vi "SmartSEM Remote API FIB Gun Valve.vi"(5 "Wait (ms)":u32=2000, 7 "Iterations":u32=3, 8 "error in":errorcluster, 10 "FIB Gun Valve":enum16{"Close", "Open"}(ring), 11 "Api":refnum<k7>(container)) -> (0 "error out":errorcluster, 3 "Api out":refnum<k7>)   [LabVIEW 2018]
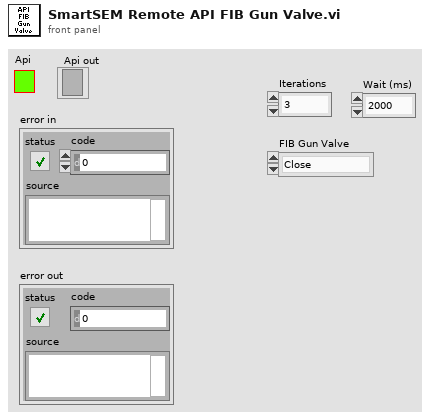
[diagram p1: front panel]
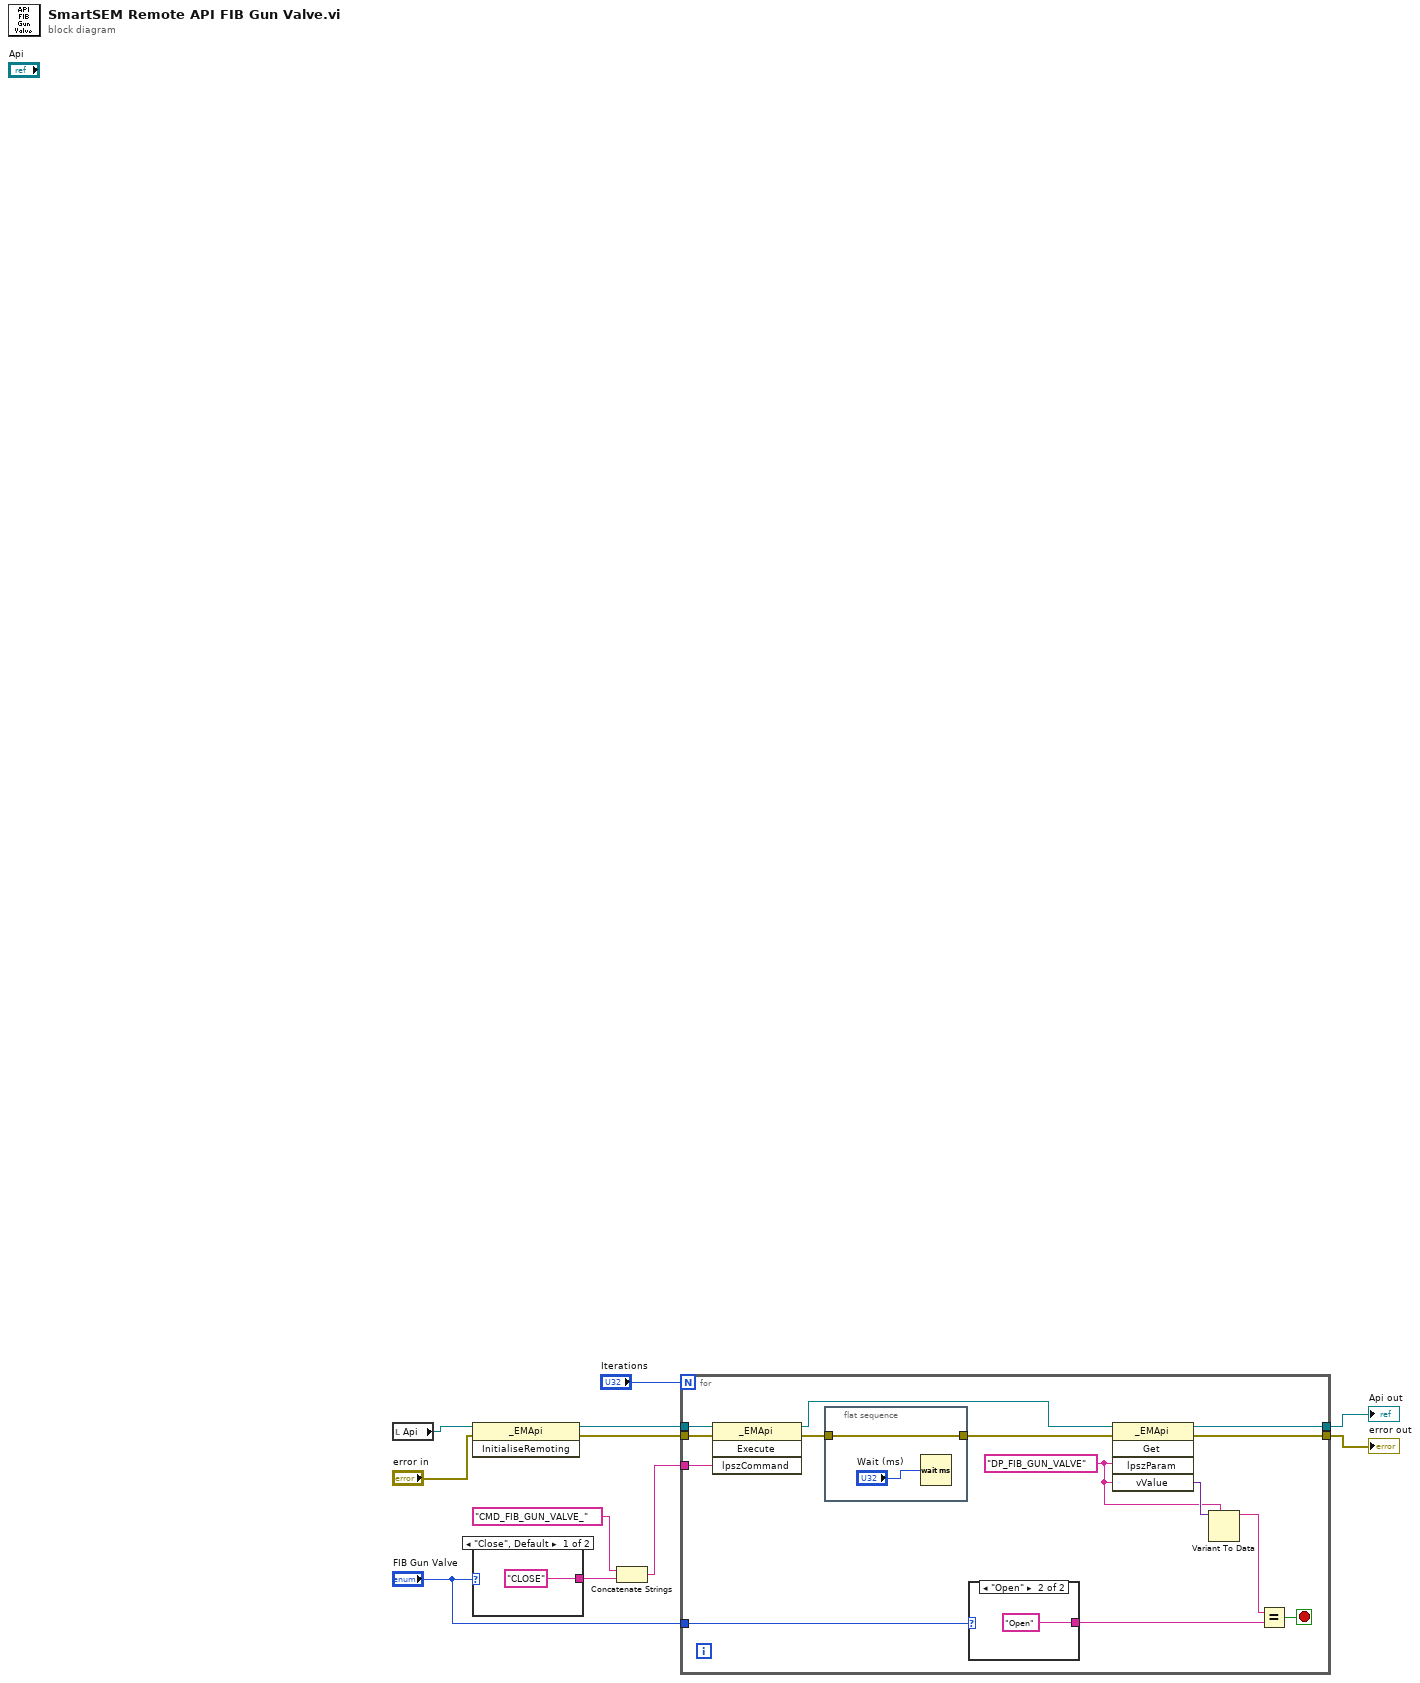
[diagram p0: block diagram]
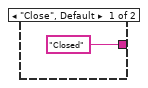
[diagram p2: hidden frame]
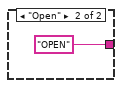
[diagram p3: hidden frame]
diagram:
  n1 = local read "Api"() -> (w11:refnum<k7>)
  n2 = invoke class="_EMApi" method="InitialiseRemoting"(reference=w11, error in="error in") -> (reference out=w10:refnum<k7>, error out=w5:errorcluster)  [unwired: 1 in, 1 out]
  n3 = case shown="\"Close\", Default" "FIB Gun Valve" {
    tunnel: ["CLOSE" ("lpszCommand") "OPEN" ("lpszCommand")] -> w8
    frame "Close", Default {
    }
    frame "Open" {
    }
  }
  n4 = Concatenate Strings("CMD_FIB_GUN_VALVE_" ("lpszCommand"), w8) -> (w7:string)
  n5 = for {
    N: "Iterations" -> [_]
    tunnel: w10 -> [w27]
    tunnel: w7 -> [w26]
    tunnel: "FIB Gun Valve" -> [w14]
    tunnel: w5 -> [w22]
    tunnel: [w21] -> w3
    tunnel: [w20] -> w4
    stop <- w23 stop-if-true
    w17 = "DP_FIB_GUN_VALVE" ("lpszParam")
    n6 = invoke class="_EMApi" method="Execute"(reference=w27, error in=w22, "lpszCommand"=w26) -> (reference out=w25:refnum<k7>, error out=w19:errorcluster)  [unwired: 1 in, 2 out]
    n7 = flat-sequence {
      tunnel: [w31] -> w18
      tunnel: w19 -> [w31]
      frame #0 {
        n8 = Wait (ms)(milliseconds to wait="Wait (ms)") -> ()  [unwired: 1 out]
      }
    }
    n9 = case shown="\"Open\"" w14 {
      tunnel: ["Closed" ("lpszCommand") "Open" ("lpszCommand")] -> w16
      frame "Close", Default {
      }
      frame "Open" {
      }
    }
    n10 = invoke class="_EMApi" method="Get"(reference=w25, error in=w18, "lpszParam"=w17, "vValue"=w17) -> (reference out=w21:refnum<k7>, error out=w20:errorcluster, "vValue"=w24:variant)  [unwired: 1 in, 2 out]
    n11 = Variant To Data(type=w17, Variant=w24) -> (data=w15:string)  [unwired: 1 in, 1 out]
    n12 = Equal?(x=w15, y=w16) -> (x = y?=w23:bool)
  }
  "Api out" <- w3
  "error out" <- w4
